vi "Configuration Keys.vi"(8 "error in":errorcluster, 11 "6032A in":refnum<class "6032A.lvclass">) -> (0 "error out":errorcluster, 2 "Required Keys":string[](array[string]), 3 "6032A out":refnum<class "6032A.lvclass">)   [LabVIEW 2019, in "6032A.lvlib" / "6032A.lvclass"]
doc: "Configuration Keys is a dynamic dispatch VI that reads a full inheritance chain's required key list.\n\nThis means each instrument must override this vi, and call the parent method . The end result is a comprehensive list of required keys that must be present in an instrument's config.ini file to correctly function."
uses:
  Library/6032A.lvclass
  Custom Controls/Configuration Keys.ctl
  builds/Instruments/PowerSupply.lvlibp/Library/PowerSupply.lvclass
panel:
  in  "Configuration Keys":T1
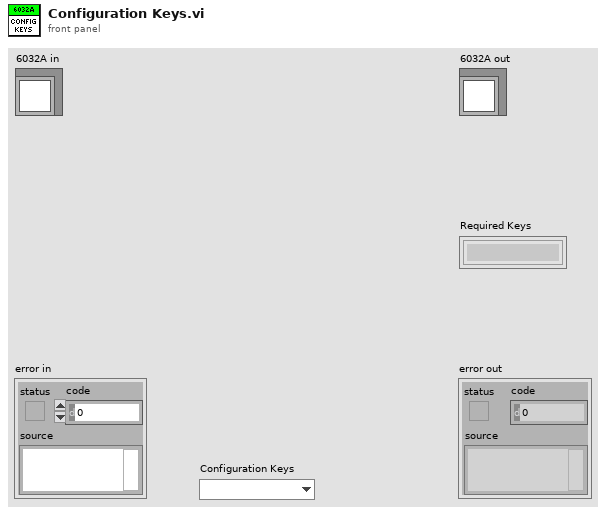
[diagram p1: front panel]
types:
  T1 = typedef "6032A.lvlib/6032A.lvclass/Configuration Keys.ctl" = enum16{""}
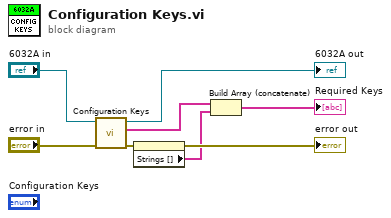
[diagram p0: block diagram]
diagram:
  n1 = call-parent "Configuration Keys.vi"("error in"="error in", "PowerSupply in"="6032A in") -> ("error out"=w5:errorcluster, "Required Keys"=w2:string[], "PowerSupply out"=→"6032A out":refnum<class "6032A.lvclass">)  [unwired: 7 in]
  n2 = property on="Configuration Keys" class="Enum (strict)"(error in=w5) -> (error out=→"error out":errorcluster, "Strings []"=w3:string[])  [unwired: 1 in, 1 out]
  n3 = Build Array (concatenate)(w2, w3) -> (→"Required Keys":string[])
